vi "get selected date info.vi"(8 "error in":errorcluster, 11 "Cluster in":T1={"Running VI"=refnum, "Test VI"=refnum, "Q Ref"=refnum, "UE"=refnum, "Data"=variant, "Timeout"=-1, "ListBox[]"=[], "Source Path"=path "", "Delta Time"=0.0, "ExifInfo[]"=[], "ListIndex"=0, "counter"=0, "Format"=enum."Files Only", "total"=0, "Operation"=enum."Read Info", "Status"=""} {"ExifInfo[]"."New DateTime" format="%<%.3X>T"; "ExifInfo[]"."DateTimeOrginal" format="%<%.3X>T"}) -> (0 "error out":errorcluster, 3 "Cluster out":T1={"Running VI"=refnum, "Test VI"=refnum, "Q Ref"=refnum, "UE"=refnum, "Data"=variant, "Timeout"=-1, "ListBox[]"=[], "Source Path"=path "", "Delta Time"=0.0, "ExifInfo[]"=[], "ListIndex"=0, "counter"=0, "Format"=enum."Files Only", "total"=0, "Operation"=enum."Read Info", "Status"=""} {"ExifInfo[]"."New DateTime" format="%<%.3X>T"; "ExifInfo[]"."DateTimeOrginal" format="%<%.3X>T"}, 4 "DateTimeOrginal":timestamp)   [LabVIEW 2023, in "EXIF Modifier.lvlib"]
uses:
  Controls/exif_consumer cluster.ctl
  Controls/exif_info cluster.ctl
  EXIF Modifier.lvlib
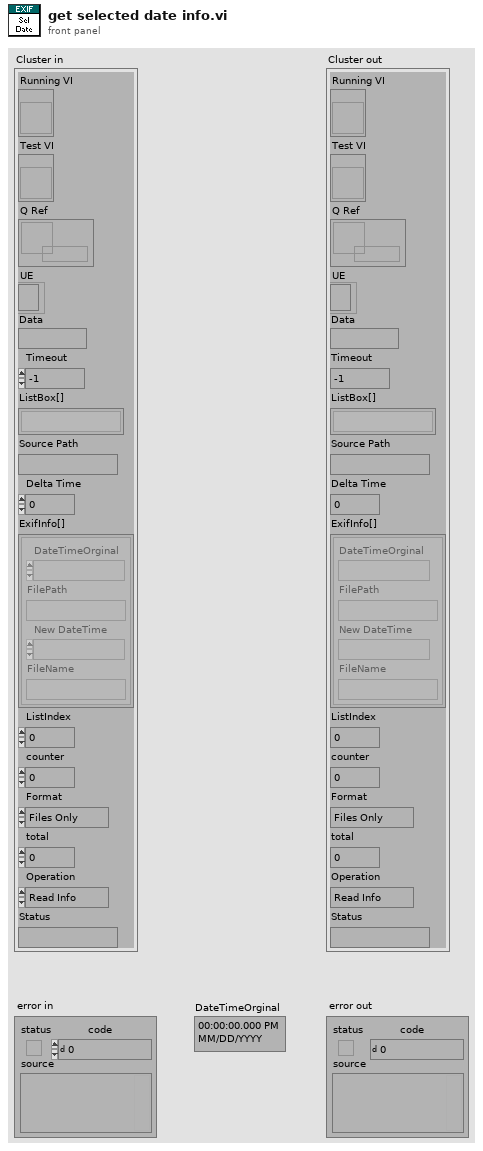
[diagram p1: front panel]
types:
  T1 = typedef "EXIF Modifier.lvlib/exif_consumer cluster.ctl" = cluster{"Running VI":refnum<vi>, "Test VI":refnum<vi>, "Q Ref":refnum<queue>, "UE":refnum<event-registration>, "Data":variant, "Timeout":i32, "ListBox[]":string[][], "Source Path":path, "Delta Time":dbl, "ExifInfo[]":T2[], "ListIndex":i32, "counter":i32, "Format":enum16{"Files Only", "Files Date", "All"}, "total":i32, "Operation":enum16{"Read Info", "Write Info"}, "Status":string}
  T2 = typedef "EXIF Modifier.lvlib/exif_info cluster.ctl" = cluster{"DateTimeOrginal":timestamp, "FilePath":path, "New DateTime":timestamp, "FileName":string}
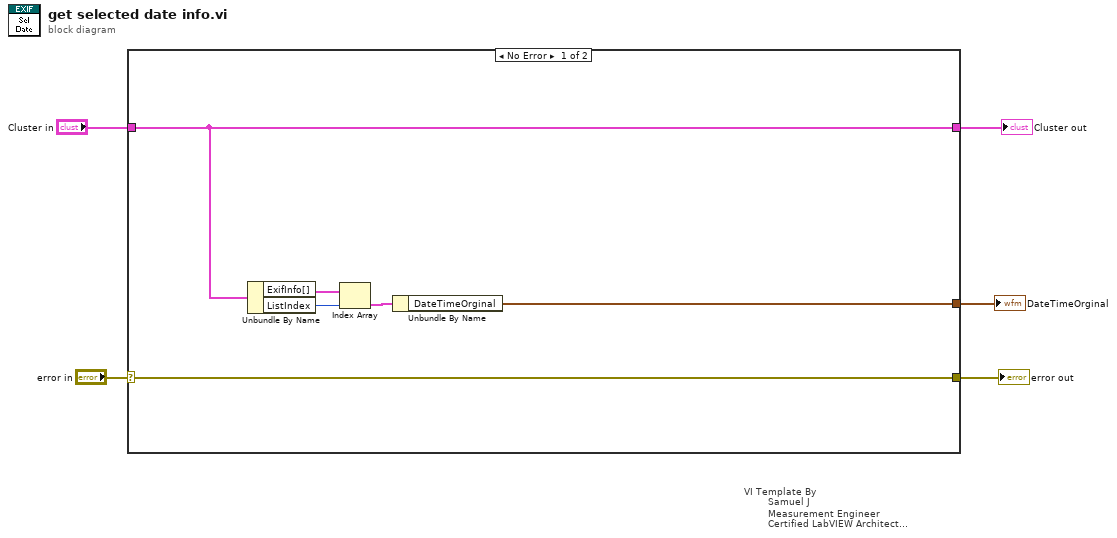
[diagram p0: block diagram]
diagram:
  n1 = case "VI Template By\n        Samuel J\n        Measurement Engineer\n        Certified LabVIEW Architect\n        Vestas Technology R&D Chennai" shown="No Error" "error in" {
    selector: "error in" -> [w11 w13]
    tunnel: [w11 w13] -> w4
    tunnel: [w7 w12] -> w2
    tunnel: "Cluster in" -> [w7 w12]
    tunnel: [w6 _] -> w1
    frame No Error {
      n2 = Unbundle By Name(w7) -> ("ExifInfo[]"=w9:T2[], "ListIndex"=w10:i32)
      n3 = Index Array(array=w9, index=w10) -> (element=w8:T2)
      n4 = Unbundle By Name(w8) -> ("DateTimeOrginal"=w6:timestamp)
    }
    frame Error {
    }
  }
  "error out" <- w4
  "Cluster out" <- w2
  "DateTimeOrginal" <- w1
